vi "test-unscented-kalman-filter-test2-callback-func-f.vi"(9 "U":T1, 10 "X":T1, 11 "Info":variant) -> (0 "Error":bool, 3 "XDOT":T1)   [LabVIEW 2019]
uses:
  <vilib>/Analysis/Matrix/Datatypes/RealMatrix.ctl
  <vilib>/Analysis/NI_AALBase.lvlib
  <vilib>/Analysis/baseanly.llb/Real A x B.vi
  <vilib>/Analysis/Matrix/NI_Matrix.lvlib
  <vilib>/Analysis/Matrix/Numeric/Add/Add - RM,RM.vi
panel:
  in  "Cluster":cluster{"A":T1, "B":T1}
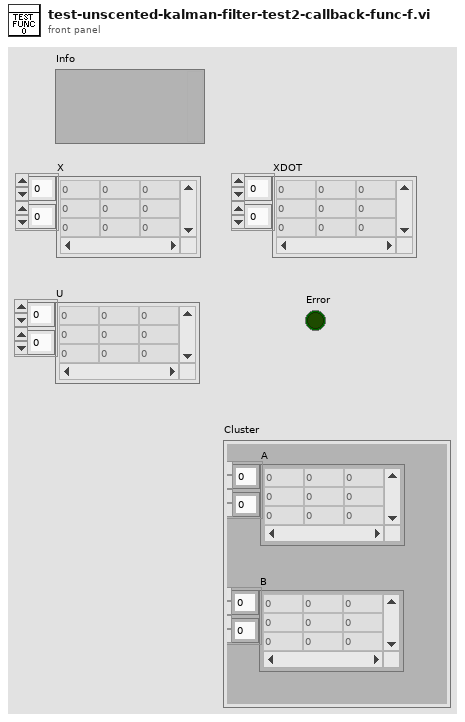
[diagram p1: front panel]
types:
  T1 = typedef "NI_Matrix.lvlib/RealMatrix.ctl" = dbl[][]
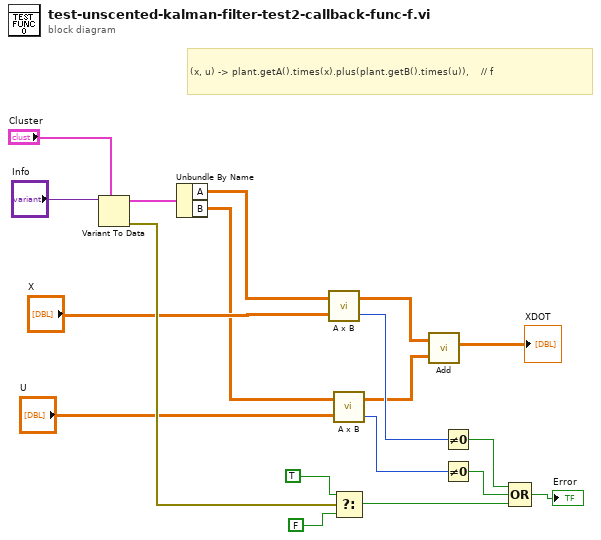
[diagram p0: block diagram]
diagram:
  # "(x, u) -> plant.getA().times(x).plus(plant.getB().times(u)),    // f"
  n1 = Variant To Data(type="Cluster", Variant="Info") -> (data=w17:cluster{"A":T1, "B":T1}, error out=w12:errorcluster)  [unwired: 1 in]
  n2 = Unbundle By Name(w17) -> ("A"=w11:T1, "B"=w9:T1)
  n3 = call-poly <vilib>:"A x B.vi"("B"="X", "A"=w11) -> ("error"=w6:i32, "A x B"=w3:T1)
  n4 = call-poly <vilib>:"A x B.vi"("B"="U", "A"=w9) -> ("error"=w7:i32, "A x B"=w2:T1)
  n5 = Select(t=TRUE, s=w12, f=FALSE) -> (s? t:f=w15:bool)
  n6 = call-poly <vilib>:"Add.vi"("Real Matrix B"=w2, "Real Matrix A"=w3) -> ("A + B"=→"XDOT":T1)
  n7 = Not Equal To 0?(x=w6) -> (x != 0?=w4:bool)
  n8 = Not Equal To 0?(x=w7) -> (x != 0?=w5:bool)
  n9 = Compound Arithmetic op=OR(w4, w5, w15) -> (→"Error":bool)
